vi "FATEK-Request Message Format.vi"(8 "error in":errorcluster, 11 "Request Message Format":T1={"Slave Station No"="01", "Command Code"=72, "Control Code"=variant} {"Command Code" items=["Read multiple data of consecutive registers"=70, "Write to multiple consecutive registers"=71]}) -> (0 "error out":errorcluster, 2 "Bytes To Read":i32, 3 "Request Message":string)   [LabVIEW 2018]
uses:
  Data Def/FATEK-Request Message Format.ctl
  Data Def/FATEK-Command Code.ctl
  Data Def/FATEK-Read multiple data of consecutive registers.ctl
  Data Def/FATEK-Write to multiple consecutive registers.ctl
  Data Def/FATEK-Device Code.ctl
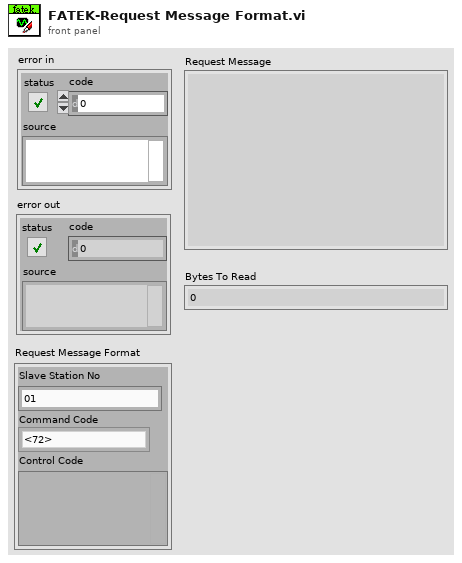
[diagram p1: front panel]
types:
  T1 = typedef "FATEK-Request Message Format.ctl" = cluster{"Slave Station No":string, "Command Code":T2, "Control Code":variant}
  T2 = typedef "FATEK-Command Code.ctl" = u16
  T3 = typedef "FATEK-Read multiple data of consecutive registers.ctl" = cluster{"Number N":u8, "Device Code":enum16{"X", "Y", "M", "R", "D"}, "Start Position":u16}
  T4 = typedef "FATEK-Write to multiple consecutive registers.ctl" = cluster{"Number N":u8, "Device Code":T5, "Position":u16, "Value":i16[]}
  T5 = typedef "FATEK-Device Code.ctl" = enum16{"X", "Y", "M", "R", "D"}
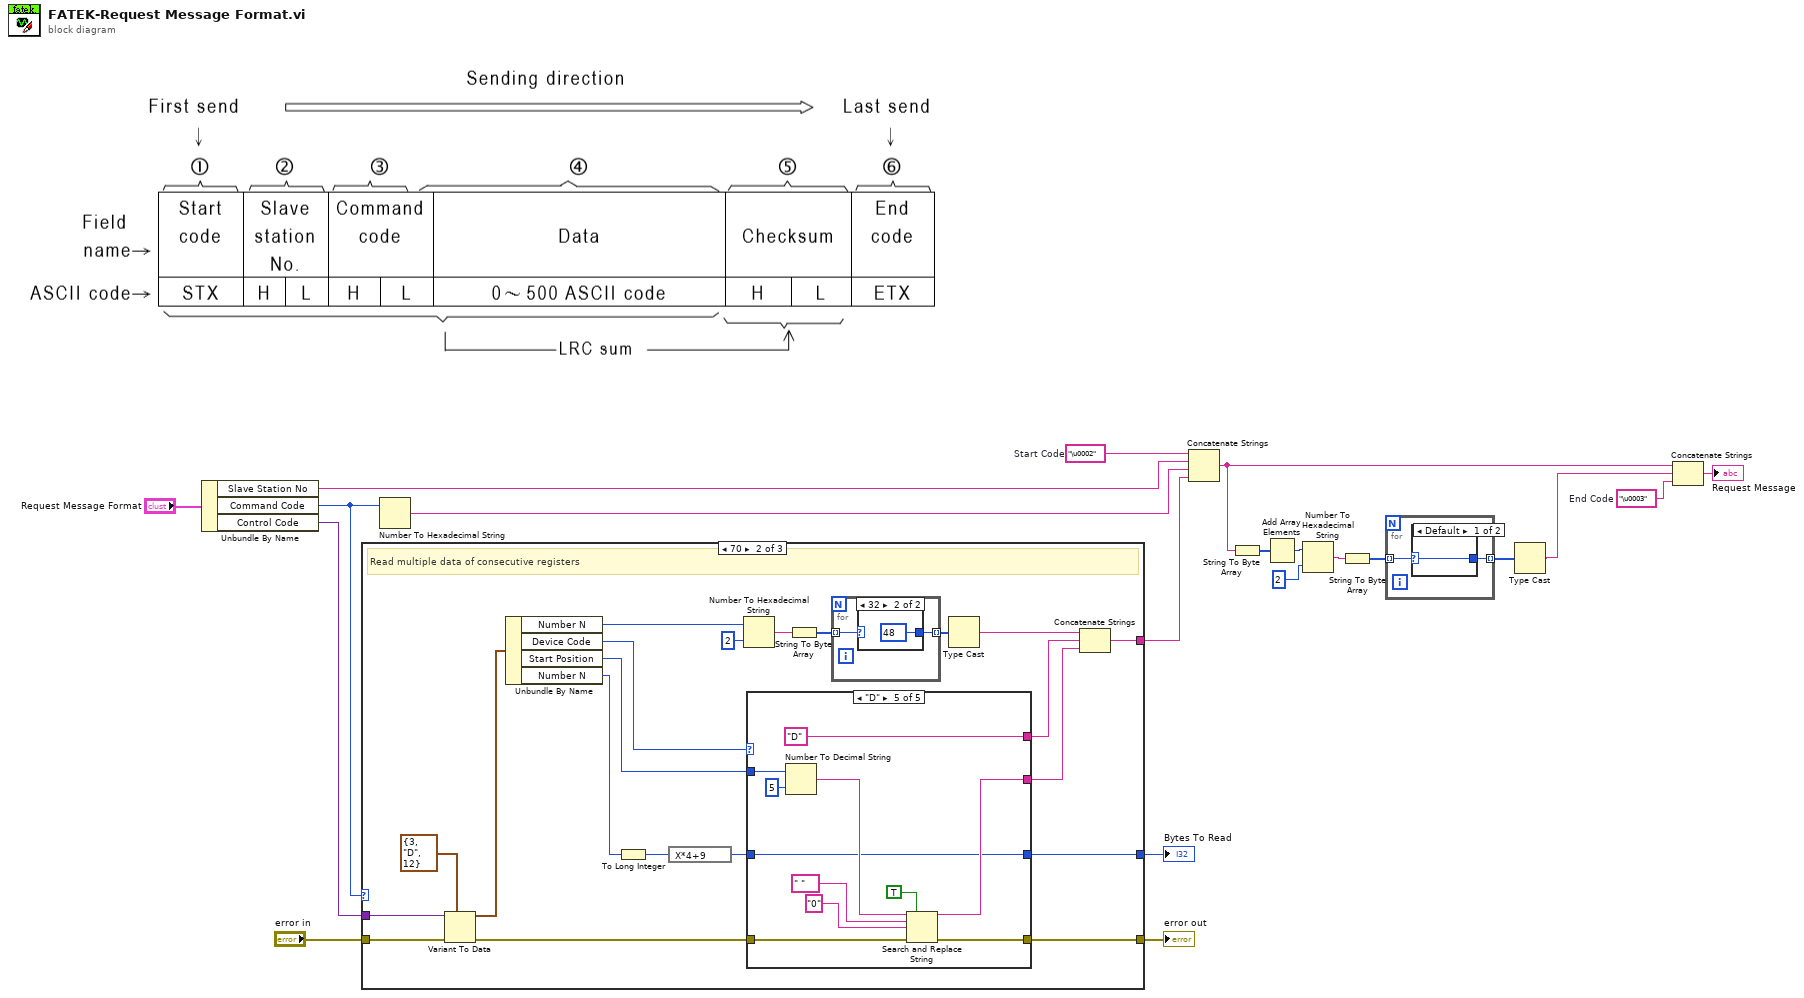
[diagram p0: block diagram]
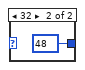
[diagram p2: hidden frame]
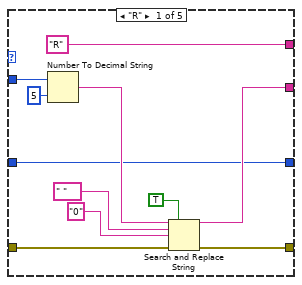
[diagram p4: hidden frame]
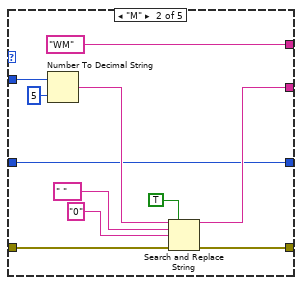
[diagram p5: hidden frame]
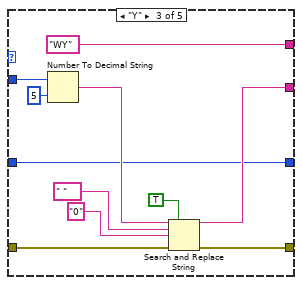
[diagram p6: hidden frame]
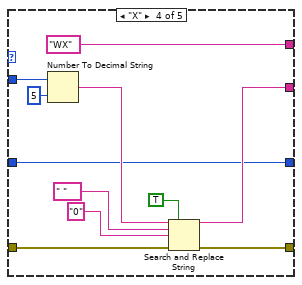
[diagram p7: hidden frame]
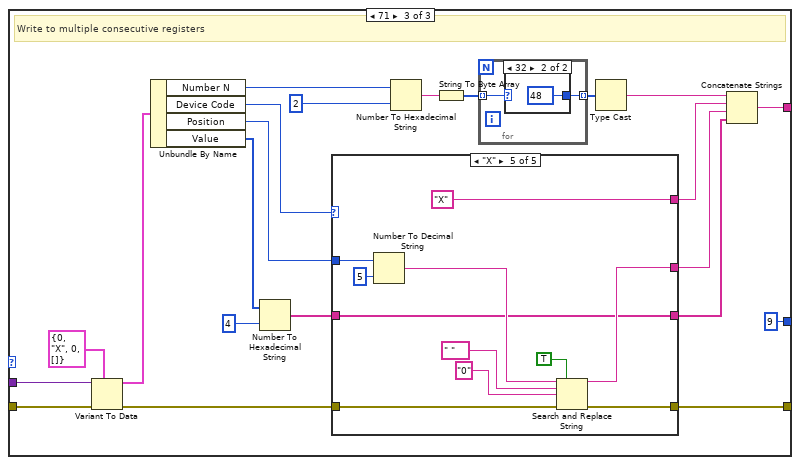
[diagram p9: hidden frame]
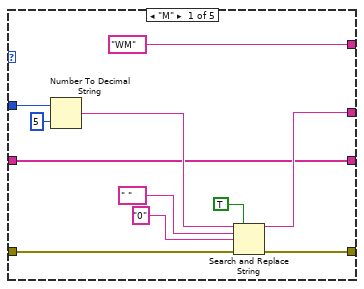
[diagram p10: hidden frame]
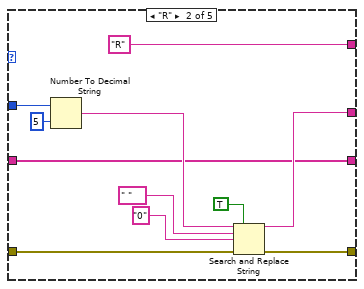
[diagram p11: hidden frame]
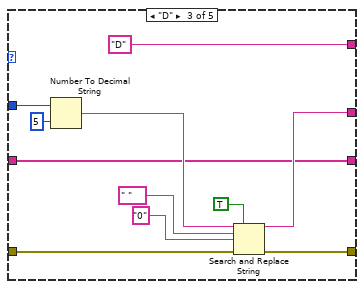
[diagram p12: hidden frame]
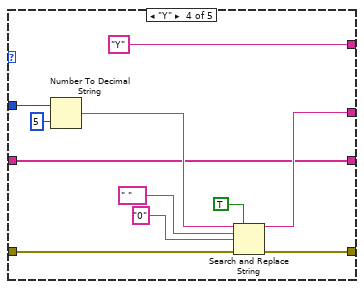
[diagram p13: hidden frame]
diagram:
  w11 = "\u0003"  # End Code
  w19 = "\u0002"  # Start Code
  n1 = Unbundle By Name("Request Message Format") -> ("Slave Station No"=w18:string, "Command Code"=w14:T2, "Control Code"=w17:variant)
  n2 = case shown="70" w14 {
    tunnel: w17 -> [_ w41 w122]
    tunnel: [_ w40 w121] -> w15
    tunnel: "error in" -> [w21 w42 w123]
    tunnel: [w21 w24 w104] -> w8
    tunnel: [_ w22 9] -> w1
    frame Default {
      # "Null"
    }
    frame 70 {
      # "Read multiple data of consecutive registers"
      n3 = Variant To Data(error in=w42, type=T3 {"Number N"=3, "Device Code"=enum."D", "Start Position"=12} ("Read multiple data of consecutive registers"), Variant=w41) -> (data=w32:T3, error out=w25:errorcluster)
      n4 = Unbundle By Name(w32) -> ("Number N"=w39:u8, "Device Code"=w31:enum16{"X", "Y", "M", "R", "D"}, "Start Position"=w26:u16, "Number N"=w28:u8)
      n5 = To Long Integer(number=w28) -> (32bit integer=w27:i32)
      n6 = expression code="X*4+9"(w27) -> (w23:i32)
      n7 = Number To Hexadecimal String(1:i16 2 ("width (-)"), 2:w39) -> (0:w35:string)
      n8 = case shown="\"D\"" w31 {
        tunnel: ["R" "WM" "WY" "WX" "D"] -> w30
        tunnel: w26 -> [w47 w58 w69 w80 w91]
        tunnel: [w46 w57 w68 w79 w90] -> w29
        tunnel: w25 -> [w45 w56 w67 w78 w89]
        tunnel: [w44 w55 w66 w77 w88] -> w24
        tunnel: w23 -> [w43 w54 w65 w76 w87]
        tunnel: [w43 w54 w65 w76 w87] -> w22
        frame "R" {
          n9 = Number To Decimal String(number=w47, width (-)=i16 5) -> (decimal integer string=w52:string)
          n10 = Search and Replace String(replace all?=TRUE ("replace all? (F)"), input string=w52, search string=" ", replace string="0", error in=w45) -> (result string=w46:string, error out=w44:errorcluster)  [unwired: 3 in, 2 out]
        }
        frame "M" {
          n11 = Number To Decimal String(number=w58, width (-)=i16 5) -> (decimal integer string=w63:string)
          n12 = Search and Replace String(replace all?=TRUE ("replace all? (F)"), input string=w63, search string=" ", replace string="0", error in=w56) -> (result string=w57:string, error out=w55:errorcluster)  [unwired: 3 in, 2 out]
        }
        frame "Y" {
          n13 = Number To Decimal String(number=w69, width (-)=i16 5) -> (decimal integer string=w74:string)
          n14 = Search and Replace String(replace all?=TRUE ("replace all? (F)"), input string=w74, search string=" ", replace string="0", error in=w67) -> (result string=w68:string, error out=w66:errorcluster)  [unwired: 3 in, 2 out]
        }
        frame "X" {
          n15 = Number To Decimal String(number=w80, width (-)=i16 5) -> (decimal integer string=w85:string)
          n16 = Search and Replace String(replace all?=TRUE ("replace all? (F)"), input string=w85, search string=" ", replace string="0", error in=w78) -> (result string=w79:string, error out=w77:errorcluster)  [unwired: 3 in, 2 out]
        }
        frame "D" {
          n17 = Number To Decimal String(number=w91, width (-)=i16 5) -> (decimal integer string=w96:string)
          n18 = Search and Replace String(replace all?=TRUE ("replace all? (F)"), input string=w96, search string=" ", replace string="0", error in=w89) -> (result string=w90:string, error out=w88:errorcluster)  [unwired: 3 in, 2 out]
        }
      }
      n19 = String To Byte Array(string=w35) -> (unsigned byte array=w37:u8[])
      n20 = for {
        tunnel: w37 -> [w99] mode=indexing
        tunnel: [w98] -> w36 mode=indexing
        n21 = case shown="32" w99 {
          selector: w99 -> [w100 _]
          tunnel: [w100 u8 48] -> w98
          frame Default {
          }
          frame 32 {
          }
        }
      }
      n22 = Type Cast(x=w36) -> (*(type *) &x=w34:string)  [unwired: 1 in]
      n23 = Concatenate Strings(w34, w30, w29) -> (w40:string)
    }
    frame 71 {
      # "Write to multiple consecutive registers"
      n24 = Variant To Data(error in=w123, type=T4 {"Number N"=0, "Device Code"=enum."X", "Position"=0, "Value"=[]} ("Write to multiple consecutive registers"), Variant=w122) -> (data=w114:T4, error out=w105:errorcluster)
      n25 = Unbundle By Name(w114) -> ("Number N"=w120:u8, "Device Code"=w113:T5, "Position"=w110:u16, "Value"=w108:i16[])
      n26 = Number To Hexadecimal String(1:i16 4 ("width (-)"), 2:w108) -> (0:w103:string[])
      n27 = case shown="\"X\"" w113 {
        tunnel: ["WM" "R" "D" "Y" "X"] -> w112
        tunnel: w110 -> [w132 w143 w154 w165 w176]
        tunnel: [w125 w136 w147 w158 w169] -> w111
        tunnel: w105 -> [w128 w139 w150 w161 w172]
        tunnel: [w127 w138 w149 w160 w171] -> w104
        tunnel: w103 -> [w124 w135 w146 w157 w168]
        tunnel: [w124 w135 w146 w157 w168] -> w102
        frame "M" {
          n28 = Number To Decimal String(number=w132, width (-)=i16 5) -> (decimal integer string=w126:string)
          n29 = Search and Replace String(replace all?=TRUE ("replace all? (F)"), input string=w126, search string=" ", replace string="0", error in=w128) -> (result string=w125:string, error out=w127:errorcluster)  [unwired: 3 in, 2 out]
        }
        frame "R" {
          n30 = Number To Decimal String(number=w143, width (-)=i16 5) -> (decimal integer string=w137:string)
          n31 = Search and Replace String(replace all?=TRUE ("replace all? (F)"), input string=w137, search string=" ", replace string="0", error in=w139) -> (result string=w136:string, error out=w138:errorcluster)  [unwired: 3 in, 2 out]
        }
        frame "D" {
          n32 = Number To Decimal String(number=w154, width (-)=i16 5) -> (decimal integer string=w148:string)
          n33 = Search and Replace String(replace all?=TRUE ("replace all? (F)"), input string=w148, search string=" ", replace string="0", error in=w150) -> (result string=w147:string, error out=w149:errorcluster)  [unwired: 3 in, 2 out]
        }
        frame "Y" {
          n34 = Number To Decimal String(number=w165, width (-)=i16 5) -> (decimal integer string=w159:string)
          n35 = Search and Replace String(replace all?=TRUE ("replace all? (F)"), input string=w159, search string=" ", replace string="0", error in=w161) -> (result string=w158:string, error out=w160:errorcluster)  [unwired: 3 in, 2 out]
        }
        frame "X" {
          n36 = Number To Decimal String(number=w176, width (-)=i16 5) -> (decimal integer string=w170:string)
          n37 = Search and Replace String(replace all?=TRUE ("replace all? (F)"), input string=w170, search string=" ", replace string="0", error in=w172) -> (result string=w169:string, error out=w171:errorcluster)  [unwired: 3 in, 2 out]
        }
      }
      n38 = Number To Hexadecimal String(1:i16 2 ("width (-)"), 2:w120) -> (0:w116:string)
      n39 = String To Byte Array(string=w116) -> (unsigned byte array=w118:u8[])
      n40 = for {
        tunnel: w118 -> [w180] mode=indexing
        tunnel: [w179] -> w117 mode=indexing
        n41 = case shown="32" w180 {
          selector: w180 -> [w181 _]
          tunnel: [w181 u8 48] -> w179
          frame Default {
          }
          frame 32 {
          }
        }
      }
      n42 = Type Cast(x=w117) -> (*(type *) &x=w115:string)  [unwired: 1 in]
      n43 = Concatenate Strings(w115, w112, w111, w102) -> (w121:string)
    }
  }
  "error out" <- w8
  "Bytes To Read" <- w1
  n44 = Number To Hexadecimal String(2:w14) -> (0:w16:string)  [unwired: 1 in]
  n45 = Concatenate Strings(w19, w18, w16, w15) -> (w12:string)
  n46 = String To Byte Array(string=w12) -> (unsigned byte array=w13:u8[])
  n47 = Add Array Elements(numeric array=w13) -> (sum=w6:u8)
  n48 = Number To Hexadecimal String(1:i16 2 ("width (-)"), 2:w6) -> (0:w5:string)
  n49 = String To Byte Array(string=w5) -> (unsigned byte array=w4:u8[])
  n50 = for {
    tunnel: w4 -> [w184] mode=indexing
    tunnel: [w183] -> w3 mode=indexing
    n51 = case shown="Default" w184 {
      selector: w184 -> [w185 _]
      tunnel: [w185 u8 48] -> w183
      frame Default {
      }
      frame 32 {
      }
    }
  }
  n52 = Type Cast(x=w3) -> (*(type *) &x=w2:string)  [unwired: 1 in]
  n53 = Concatenate Strings(w12, w2, w11) -> (→"Request Message":string)
